vi "Array Weighted Average.vi"(1 "Input Array":dbl[](array[numeric])) -> (0 "Weighted Average Index":dbl)   [LabVIEW 2013]
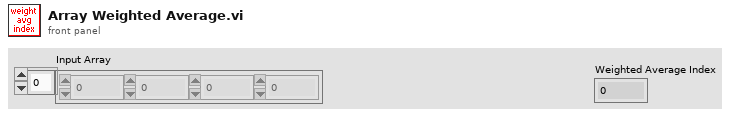
[diagram p1: front panel]
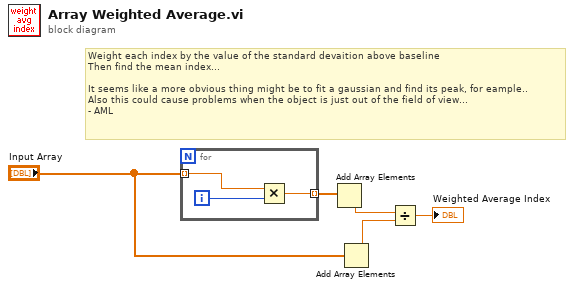
[diagram p0: block diagram]
diagram:
  # "Weight each index by the value of the standard devaition above baseline\nThen find the mean index...\n\nIt seems like a more obvious thing might be to fit a gaussian and find its peak, for eample..\nAlso this could cause problems when the object is just out of the field of view...\n- AML"
  n1 = for {
    tunnel: "Input Array" -> [w8] mode=indexing
    tunnel: [w7] -> w5 mode=indexing
    i -> [w6]
    n2 = Multiply(x=w8, y=w6) -> (x*y=w7:dbl)
  }
  n3 = Add Array Elements(numeric array=w5) -> (sum=w3:dbl)
  n4 = Add Array Elements(numeric array="Input Array") -> (sum=w2:dbl)
  n5 = Divide(x=w3, y=w2) -> (x/y=→"Weighted Average Index":dbl)
